vi "LoadServerCfg.vi"(8 "error in (no error)":errorcluster, 11 "RESTLoaderIni in":refnum<class "RESTLoaderIni.lvclass">) -> (0 "error out":errorcluster, 2 "Server config":T1={"API Root"="", "verify server"=FALSE, "Version (no version)"="", "Port (protocol specific)"=0, "Base URL"="", "Auth type"=enum."Token", "Auth string"="", "timeout (10000)"=10000}, 3 "RESTLoaderIni out":refnum<class "RESTLoaderIni.lvclass">)   [LabVIEW 2019, in "ByteREST.lvlib" / "RESTLoaderIni.lvclass"]
uses:
  RESTLoaderIni.lvclass
  LoaderBase/ServerParams.ctl
  ByteRESTClass/ByteRESTBase/Auth/Authentication_type.ctl
  RESTLoaderIni.lvclass/RESTLoaderIni.ctl
  <vilib>/Utility/config.llb/Read Key (String).vi
  <vilib>/Utility/config.llb/Write Key (String).vi
  <vilib>/Utility/config.llb/Read Key (U32).vi
  <vilib>/Utility/config.llb/Write Key (U32).vi
  <vilib>/Utility/config.llb/Read Key (I32).vi
  <vilib>/Utility/config.llb/Write Key (I32).vi
  <vilib>/Utility/config.llb/Read Key (Boolean).vi
  <vilib>/Utility/config.llb/Write Key (Boolean).vi
  <vilib>/Utility/config.llb/NI_LVConfig.lvlib
  ByteRESTClass/ByteRESTBase/RESTBase.lvclass
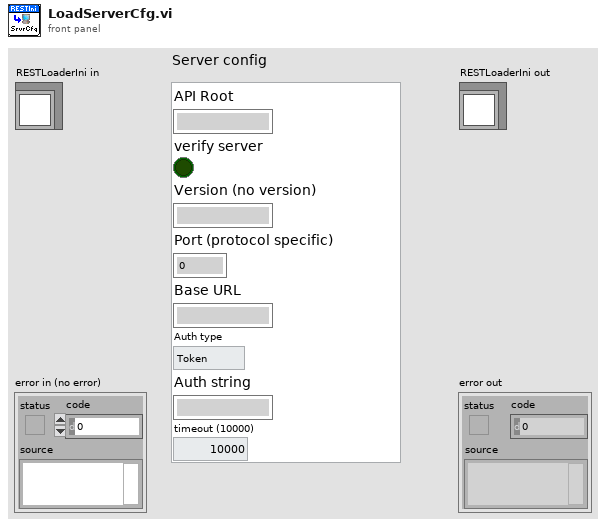
[diagram p1: front panel]
types:
  T1 = typedef "ServerParams.ctl" = cluster{"API Root":string, "verify server":bool, "Version (no version)":string, "Port (protocol specific)":u16, "Base URL":string, "Auth type":T2, "Auth string":string, "timeout (10000)":i32}
  T2 = typedef "ByteREST.lvlib/RESTBase.lvclass/Authentication_type.ctl" = enum16{"Token"}
  T3 = typedef "NI_LVConfig.lvlib/Config Data RefNum.ctl" = refnum<k1>
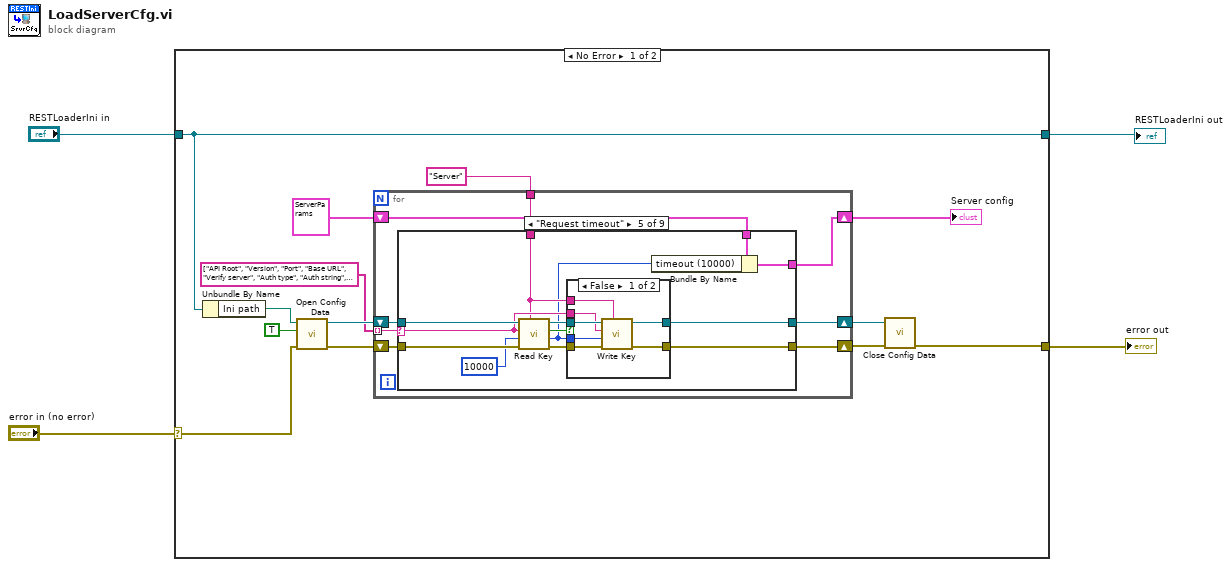
[diagram p0: block diagram]
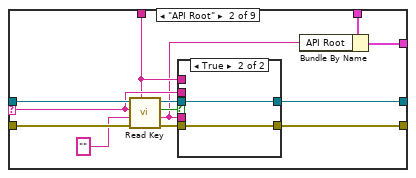
[diagram p3: hidden frame]
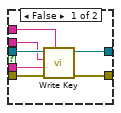
[diagram p4: hidden frame]
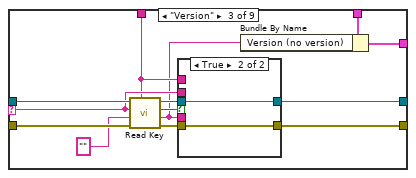
[diagram p5: hidden frame]
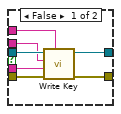
[diagram p6: hidden frame]
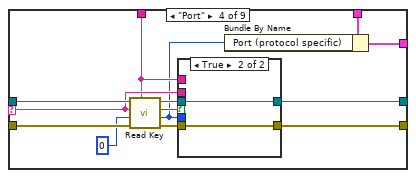
[diagram p7: hidden frame]
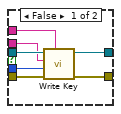
[diagram p8: hidden frame]
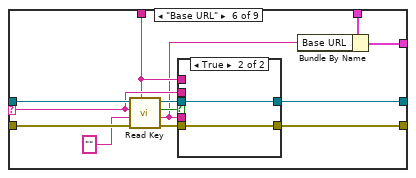
[diagram p10: hidden frame]
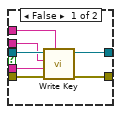
[diagram p11: hidden frame]
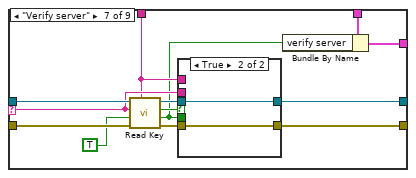
[diagram p12: hidden frame]
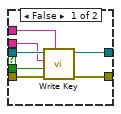
[diagram p13: hidden frame]
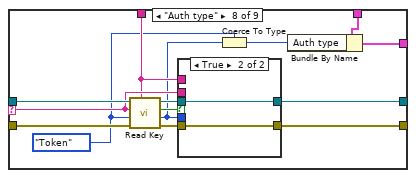
[diagram p14: hidden frame]
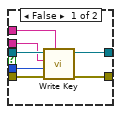
[diagram p15: hidden frame]
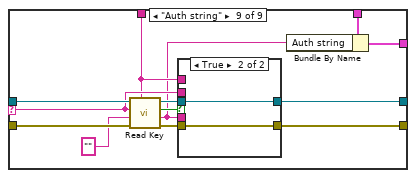
[diagram p16: hidden frame]
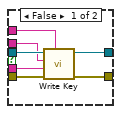
[diagram p17: hidden frame]
diagram:
  n1 = case shown="No Error" "error in (no error)" {
    selector: "error in (no error)" -> [w15 w206]
    tunnel: "RESTLoaderIni in" -> [w9 w207]
    tunnel: [w5 w206] -> w2
    tunnel: [w9 w207] -> w1
    frame No Error {
      n2 = Unbundle By Name(w9) -> ("Ini path"=w17:path)
      n3 = call <vilib>:"Open Config Data.vi"("error in (no error)"=w15, "create file if necessary (T)"=TRUE, "configuration file path"=w17) -> ("error out"=w14:errorcluster, "refnum"=w13:T3)  [unwired: 6 in, 1 out]
      n4 = for {
        tunnel: "Server" ("section") -> [w23]
        tunnel: string[] ["API Root", "Version", "Port", "Base URL", "Verify server", "Auth type", "Auth string", "Request timeout"] ("key") -> [w22] mode=indexing
        shift-right: [w20] -> w8
        shift-left: T1 {"API Root"="", "verify server"=FALSE, "Version (no version)"="", "Port (protocol specific)"=0, "Base URL"="", "Auth type"=enum."Token", "Auth string"="", "timeout (10000)"=10000} ("Server config") -> [w21]
        shift-right: [w19] -> w7
        shift-left: w14 -> [w25]
        shift-right: [w18] -> w6
        shift-left: w13 -> [w24]
        n5 = case shown="\"Request timeout\"" w22 {
          selector: w22 -> [_ w35 w57 w80 w102 w124 w146 w169 w191]
          tunnel: w25 -> [w28 w41 w63 w85 w107 w129 w151 w174 w196]
          tunnel: w24 -> [w26 w40 w62 w84 w106 w128 w150 w173 w195]
          tunnel: w23 -> [_ w34 w56 w79 w101 w123 w145 w168 w190]
          tunnel: w21 -> [w27 w33 w55 w78 w100 w122 w144 w167 w189]
          tunnel: [w27 w31 w53 w76 w98 w120 w142 w166 w188] -> w20
          tunnel: [w28 w30 w52 w75 w97 w119 w141 w165 w187] -> w19
          tunnel: [w26 w29 w51 w74 w96 w118 w140 w164 w186] -> w18
          frame Default {
          }
          frame "API Root" {
            n6 = call-poly <vilib>:"Read Key.vi"("section"=w34, "error in (no error)"=w41, "default value"="", "key"=w35, "refnum"=w40) -> ("error out"=w36:errorcluster, "value"=w32:string, "found?"=w38:bool, "refnum out"=w37:T3)  [unwired: 3 in]
            n7 = case shown="True" w38 {
              tunnel: w37 -> [w47 w49]
              tunnel: w36 -> [w48 w50]
              tunnel: w32 -> [w45 _]
              tunnel: w35 -> [w46 _]
              tunnel: w34 -> [w44 _]
              tunnel: [w43 w50] -> w30
              tunnel: [w42 w49] -> w29
              frame False {
                n8 = call-poly <vilib>:"Write Key.vi"("section"=w44, "error in (no error)"=w48, "value"=w45, "key"=w46, "refnum"=w47) -> ("error out"=w43:errorcluster, "refnum out"=w42:T3)  [unwired: 4 in, 1 out]
              }
              frame True {
              }
            }
            n9 = Bundle By Name(cluster=w33, "API Root"=w32) -> (w31:T1)
          }
          frame "Version" {
            n10 = call-poly <vilib>:"Read Key.vi"("section"=w56, "error in (no error)"=w63, "default value"="", "key"=w57, "refnum"=w62) -> ("error out"=w58:errorcluster, "value"=w54:string, "found?"=w60:bool, "refnum out"=w59:T3)  [unwired: 3 in]
            n11 = case shown="True" w60 {
              tunnel: w59 -> [w69 w71]
              tunnel: w58 -> [w70 w72]
              tunnel: w54 -> [w67 _]
              tunnel: w57 -> [w68 _]
              tunnel: w56 -> [w66 _]
              tunnel: [w65 w72] -> w52
              tunnel: [w64 w71] -> w51
              frame False {
                n12 = call-poly <vilib>:"Write Key.vi"("section"=w66, "error in (no error)"=w70, "value"=w67, "key"=w68, "refnum"=w69) -> ("error out"=w65:errorcluster, "refnum out"=w64:T3)  [unwired: 4 in, 1 out]
              }
              frame True {
              }
            }
            n13 = Bundle By Name(cluster=w55, "Version (no version)"=w54) -> (w53:T1)
          }
          frame "Port" {
            n14 = call-poly <vilib>:"Read Key.vi"("section"=w79, "error in (no error)"=w85, "default value"=u32 0, "key"=w80, "refnum"=w84) -> ("error out"=w81:errorcluster, "value"=w77:u32, "found?"=w83:bool, "refnum out"=w82:T3)  [unwired: 3 in]
            n15 = case shown="True" w83 {
              tunnel: w82 -> [w91 w93]
              tunnel: w81 -> [w92 w94]
              tunnel: w77 -> [w89 _]
              tunnel: w80 -> [w90 _]
              tunnel: w79 -> [w88 _]
              tunnel: [w87 w94] -> w75
              tunnel: [w86 w93] -> w74
              frame False {
                n16 = call-poly <vilib>:"Write Key.vi"("section"=w88, "error in (no error)"=w92, "value"=w89, "key"=w90, "refnum"=w91) -> ("error out"=w87:errorcluster, "refnum out"=w86:T3)  [unwired: 4 in, 1 out]
              }
              frame True {
              }
            }
            n17 = Bundle By Name(cluster=w78, "Port (protocol specific)"=w77) -> (w76:T1)
          }
          frame "Request timeout" {
            n18 = call-poly <vilib>:"Read Key.vi"("section"=w101, "error in (no error)"=w107, "default value"=10000, "key"=w102, "refnum"=w106) -> ("error out"=w103:errorcluster, "value"=w99:i32, "found?"=w105:bool, "refnum out"=w104:T3)  [unwired: 3 in]
            n19 = case shown="False" w105 {
              tunnel: w104 -> [w113 w115]
              tunnel: w103 -> [w114 w116]
              tunnel: w99 -> [w111 _]
              tunnel: w102 -> [w112 _]
              tunnel: w101 -> [w110 _]
              tunnel: [w109 w116] -> w97
              tunnel: [w108 w115] -> w96
              frame False {
                n20 = call-poly <vilib>:"Write Key.vi"("section"=w110, "error in (no error)"=w114, "value"=w111, "key"=w112, "refnum"=w113) -> ("error out"=w109:errorcluster, "refnum out"=w108:T3)  [unwired: 4 in, 1 out]
              }
              frame True {
              }
            }
            n21 = Bundle By Name(cluster=w100, "timeout (10000)"=w99) -> (w98:T1)
          }
          frame "Base URL" {
            n22 = call-poly <vilib>:"Read Key.vi"("section"=w123, "error in (no error)"=w129, "default value"="", "key"=w124, "refnum"=w128) -> ("error out"=w125:errorcluster, "value"=w121:string, "found?"=w127:bool, "refnum out"=w126:T3)  [unwired: 3 in]
            n23 = case shown="True" w127 {
              tunnel: w126 -> [w135 w137]
              tunnel: w125 -> [w136 w138]
              tunnel: w121 -> [w133 _]
              tunnel: w124 -> [w134 _]
              tunnel: w123 -> [w132 _]
              tunnel: [w131 w138] -> w119
              tunnel: [w130 w137] -> w118
              frame False {
                n24 = call-poly <vilib>:"Write Key.vi"("section"=w132, "error in (no error)"=w136, "value"=w133, "key"=w134, "refnum"=w135) -> ("error out"=w131:errorcluster, "refnum out"=w130:T3)  [unwired: 4 in, 1 out]
              }
              frame True {
              }
            }
            n25 = Bundle By Name(cluster=w122, "Base URL"=w121) -> (w120:T1)
          }
          frame "Verify server" {
            n26 = call-poly <vilib>:"Read Key.vi"("section"=w145, "error in (no error)"=w151, "default value"=TRUE, "key"=w146, "refnum"=w150) -> ("error out"=w147:errorcluster, "value"=w143:bool, "found?"=w149:bool, "refnum out"=w148:T3)  [unwired: 3 in]
            n27 = case shown="True" w149 {
              tunnel: w148 -> [w157 w159]
              tunnel: w147 -> [w158 w160]
              tunnel: w143 -> [w155 _]
              tunnel: w146 -> [w156 _]
              tunnel: w145 -> [w154 _]
              tunnel: [w153 w160] -> w141
              tunnel: [w152 w159] -> w140
              frame False {
                n28 = call-poly <vilib>:"Write Key.vi"("section"=w154, "error in (no error)"=w158, "value"=w155, "key"=w156, "refnum"=w157) -> ("error out"=w153:errorcluster, "refnum out"=w152:T3)  [unwired: 4 in, 1 out]
              }
              frame True {
              }
            }
            n29 = Bundle By Name(cluster=w144, "verify server"=w143) -> (w142:T1)
          }
          frame "Auth type" {
            w161 = Authentication_type."Token" ("Auth type")
            n30 = call-poly <vilib>:"Read Key.vi"("section"=w168, "error in (no error)"=w174, "default value"=w161, "key"=w169, "refnum"=w173) -> ("error out"=w170:errorcluster, "value"=w163:u32, "found?"=w172:bool, "refnum out"=w171:T3)  [unwired: 3 in]
            n31 = case shown="True" w172 {
              tunnel: w171 -> [w180 w182]
              tunnel: w170 -> [w181 w183]
              tunnel: w163 -> [w178 _]
              tunnel: w169 -> [w179 _]
              tunnel: w168 -> [w177 _]
              tunnel: [w176 w183] -> w165
              tunnel: [w175 w182] -> w164
              frame False {
                n32 = call-poly <vilib>:"Write Key.vi"("section"=w177, "error in (no error)"=w181, "value"=w178, "key"=w179, "refnum"=w180) -> ("error out"=w176:errorcluster, "refnum out"=w175:T3)  [unwired: 4 in, 1 out]
              }
              frame True {
              }
            }
            n33 = Coerce To Type(0:w163, 1:w161) -> (2:w162:T2)
            n34 = Bundle By Name(cluster=w167, "Auth type"=w162) -> (w166:T1)
          }
          frame "Auth string" {
            n35 = call-poly <vilib>:"Read Key.vi"("section"=w190, "error in (no error)"=w196, "default value"="", "key"=w191, "refnum"=w195) -> ("error out"=w192:errorcluster, "value"=w184:string, "found?"=w194:bool, "refnum out"=w193:T3)  [unwired: 3 in]
            n36 = case shown="True" w194 {
              tunnel: w193 -> [w202 w204]
              tunnel: w192 -> [w203 w205]
              tunnel: w184 -> [w200 _]
              tunnel: w191 -> [w201 _]
              tunnel: w190 -> [w199 _]
              tunnel: [w198 w205] -> w187
              tunnel: [w197 w204] -> w186
              frame False {
                n37 = call-poly <vilib>:"Write Key.vi"("section"=w199, "error in (no error)"=w203, "value"=w200, "key"=w201, "refnum"=w202) -> ("error out"=w198:errorcluster, "refnum out"=w197:T3)  [unwired: 4 in, 1 out]
              }
              frame True {
              }
            }
            n38 = Bundle By Name(cluster=w189, "Auth string"=w184) -> (w188:T1)
          }
        }
      }
      "Server config" <- w8
      n39 = call <vilib>:"Close Config Data.vi"("error in (no error)"=w7, "refnum"=w6) -> ("error out"=w5:errorcluster)  [unwired: 8 in, 1 out]
    }
    frame Error {
    }
  }
  "error out" <- w2
  "RESTLoaderIni out" <- w1
